vi "Highlight Selected Row.vi"(8 "error in (no error)":errorcluster caption="错误输入（无错误）", 9 "Origin BK Color":u32(colorbox)=16448250, 10 "BK Color In":u32(colorbox)=11776947, 11 "Table Ref In":refnum<vi>) -> (0 "error out":errorcluster caption="错误输出", 3 "Table Ref Out":refnum<vi>)   [LabVIEW 2013, in "Table Tool.lvlib"]
uses:
  Table Tool.lvlib
  Custum Type/GetOrSet.ctl
  Property/Set Or get ActiveCell Bk Color.vi
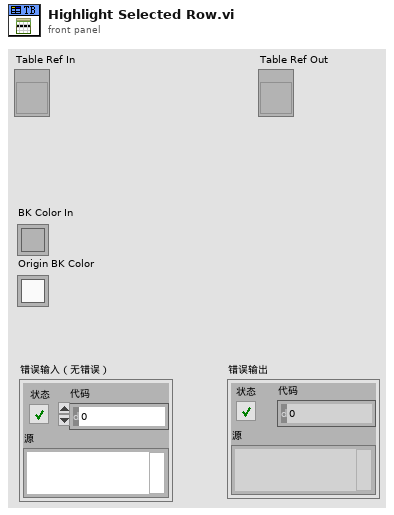
[diagram p1: front panel]
types:
  T1 = typedef "Table Tool.lvlib/GetOrSet.ctl" = enum16{"Get", "Set"}
  T2 = typedef "LVRowAndColumnTypeDef.ctl" = cluster{"Row":i32, "Column":i32}
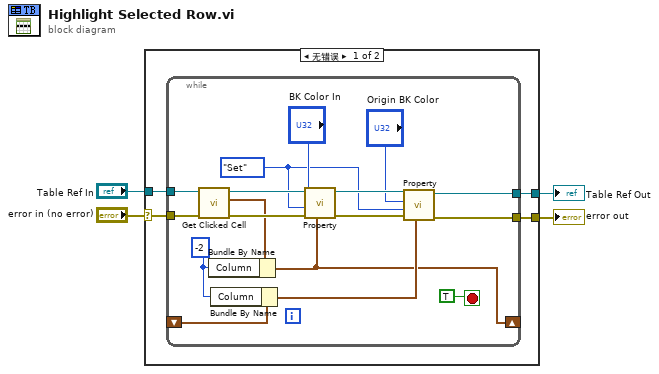
[diagram p0: block diagram]
diagram:
  n1 = case shown="无错误" "error in (no error)" {
    selector: "error in (no error)" -> [w7 w27]
    tunnel: "Table Ref In" -> [w8 w26]
    tunnel: [w5 w26] -> w2
    tunnel: [w6 w27] -> w1
    frame No Error {
      n2 = while {
        tunnel: w8 -> [w24]
        tunnel: w7 -> [w23]
        shift-right: [w9] -> _
        shift-left: _ -> [w18]
        tunnel: [w11] -> w6
        tunnel: [w10] -> w5
        stop <- TRUE stop-if-true
        w13 = GetOrSet."Set" ("Mode")
        w17 = -2 ("Column")
        n3 = call "Get Clicked Cell.vi"("error in (no error)"=w23, "Table Ref In"=w24) -> ("error out"=w22:errorcluster, "Clicked Cell"=w20:T2, "Table Ref Out"=w21:refnum<vi>)  [unwired: 7 in]
        n4 = Bundle By Name(cluster=w20, "Column"=w17) -> (w9:T2)
        n5 = Bundle By Name(cluster=w18, "Column"=w17) -> (w12:T2)
        n6 = call-poly "Property.vi"("Active Cell"=w9, "error in (no error)"=w22, "Mode"=w13, "BK Color In"="BK Color In", "Table Ref In"=w21) -> ("error out"=w16:errorcluster, "Table Ref Out"=w15:refnum<vi>)  [unwired: 4 in, 1 out]
        n7 = call-poly "Property.vi"("Active Cell"=w12, "error in (no error)"=w16, "Mode"=w13, "BK Color In"="Origin BK Color", "Table Ref In"=w15) -> ("error out"=w11:errorcluster, "Table Ref Out"=w10:refnum<vi>)  [unwired: 4 in, 1 out]
      }
    }
    frame Error {
    }
  }
  "Table Ref Out" <- w2
  "error out" <- w1
